vi "Json to Error decoder.vi"(8 "error in":errorcluster, 11 "body":string) -> (0 "error out":errorcluster)   [LabVIEW 2019, in "firebase.lvclass"]
uses:
  firebase.lvclass
  d4c846f1-14f9-4301-baca-c4c48552c76e.vi
  Error Message--cluster.ctl
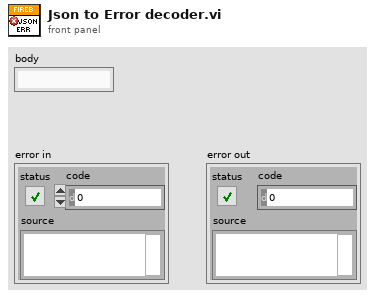
[diagram p1: front panel]
types:
  T1 = typedef "firebase.lvclass/Error Message--cluster.ctl" = cluster{"error":cluster{"code":i32, "message":string, "errors":cluster{"message":string, "domain":string, "reason":string}[]}}
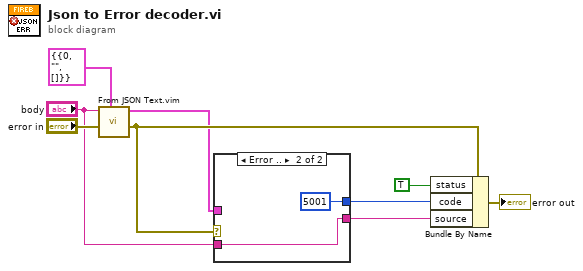
[diagram p0: block diagram]
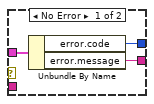
[diagram p2: hidden frame]
diagram:
  n1 = call "From JSON Text.vim"("Data Type and Default Value"=T1 {"error"={"code"=0, "message"="", "errors"=[]}} ("Error Message"), "error in (no error)"="error in", "JSON"="body") -> ("error out"=w7:errorcluster, "Data out"=w3:T1)  [unwired: 7 in]
  n2 = case shown="Error .." w7 {
    tunnel: [w12 w14] -> w5
    tunnel: [w11 5001 ("code")] -> w4
    tunnel: w3 -> [w10 _]
    tunnel: "body" -> [_ w14]
    frame No Error {
      n3 = Unbundle By Name(w10) -> ("error.code"=w11:i32, "error.message"=w12:string)
    }
    frame Error {
    }
  }
  n4 = Bundle By Name(cluster=w7, "status"=TRUE, "code"=w4, "source"=w5) -> (→"error out":errorcluster)
